vi "Set parameters.vi"(8 "error in (no error)":errorcluster caption="entrée d'erreur (pas d'erreur)", 11 "DelayLineSimulation en entrée":refnum<class "DelayLineEmulate.lvclass">) -> (0 "error out":errorcluster caption="sortie d'erreur", 3 "DelayLineSimulation en sortie":refnum<class "DelayLineEmulate.lvclass">)   [LabVIEW 2015, in "DelayLineEmulate.lvclass"]
uses:
  DelayLineEmulate.lvclass
  GeneralFunctionality/GeneralFunctionality.lvclass/GeneralFunctionality.ctl
  DelayLine.lvclass/DelayLine.ctl
  Config/Config.lvclass
  GeneralFunctionality/GeneralFunctionality.lvclass
  DelayLine.lvclass
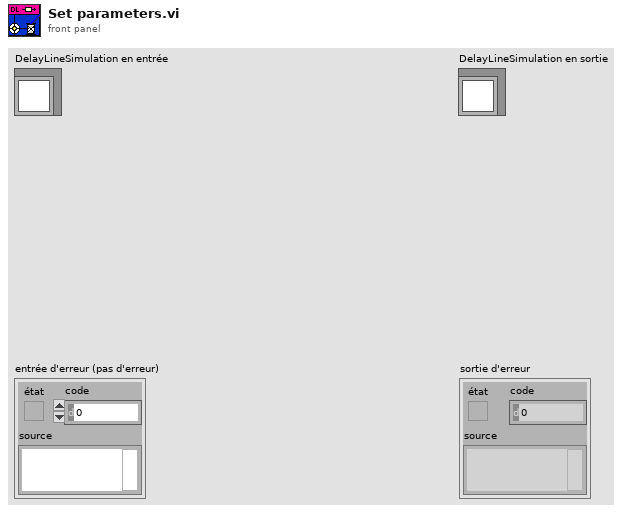
[diagram p1: front panel]
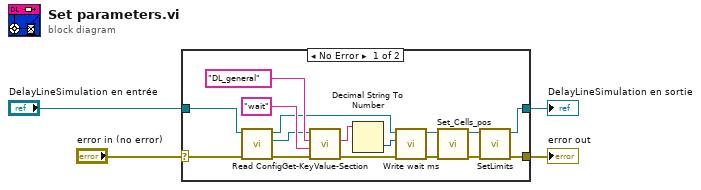
[diagram p0: block diagram]
diagram:
  n1 = case shown="No Error" "error in (no error)" {
    selector: "error in (no error)" -> [w12 w21]
    tunnel: [w7 w22] -> w1
    tunnel: "DelayLineSimulation en entrée" -> [w13 w22]
    tunnel: [w6 w21] -> w2
    frame No Error {
      n2 = call "Read Config.vi"("error in (no error)"=w12, "GeneralFunctionality en entrée"=w13) -> ("error out"=w20:errorcluster, "Config.lvclass"=w17:refnum<class "Config.lvclass">, "GeneralFunctionality en sortie"=w5:refnum<class "DelayLineEmulate.lvclass">)  [unwired: 7 in]
      n3 = call-dynamic "Get-KeyValue-Section.vi"("error in (no error)"=w20, "Key"="wait", "Section"="DL_general", "Config in"=w17) -> ("error out"=w15:errorcluster, "Value"=w16:string)  [unwired: 5 in, 1 out]
      n4 = Decimal String To Number(string=w16) -> (number=w14:i32)  [unwired: 2 in, 1 out]
      n5 = call "Write wait ms.vi"("error in (no error)"=w15, "wait ms"=w14, "DelayLine in"=w5) -> ("error out"=w11:errorcluster, "DelayLine out"=w10:refnum<class "DelayLineEmulate.lvclass">)  [unwired: 7 in]
      n6 = call "Set_Cells_pos.vi"("error in (no error)"=w11, "DelayLine in"=w10) -> ("error out"=w9:errorcluster, "DelayLine out"=w8:refnum<class "DelayLineEmulate.lvclass">)  [unwired: 8 in]
      n7 = call "SetLimits.vi"("error in (no error)"=w9, "DelayLineEmulate in"=w8) -> ("error out"=w6:errorcluster, "DelayLineEmulate out"=w7:refnum<class "DelayLineEmulate.lvclass">)  [unwired: 8 in]
    }
    frame Error {
    }
  }
  "error out" <- w2
  "DelayLineSimulation en sortie" <- w1
